vi "AudioTest.Compare Plot to Limit, Get Margin.vi"(8 "error in (no error)":errorcluster, 10 "Plot Limit":T1, 11 "Plot Data":T1) -> (0 "error out":errorcluster, 3 "Margin":dbl)   [LabVIEW 2018]
uses:
  TypeDefs/AudioTest.Result Plot Data.ctl
panel:
  out "Freq":dbl
  out "XY Graph":cluster{"X":dbl[], "Y":dbl[]}[](graph)
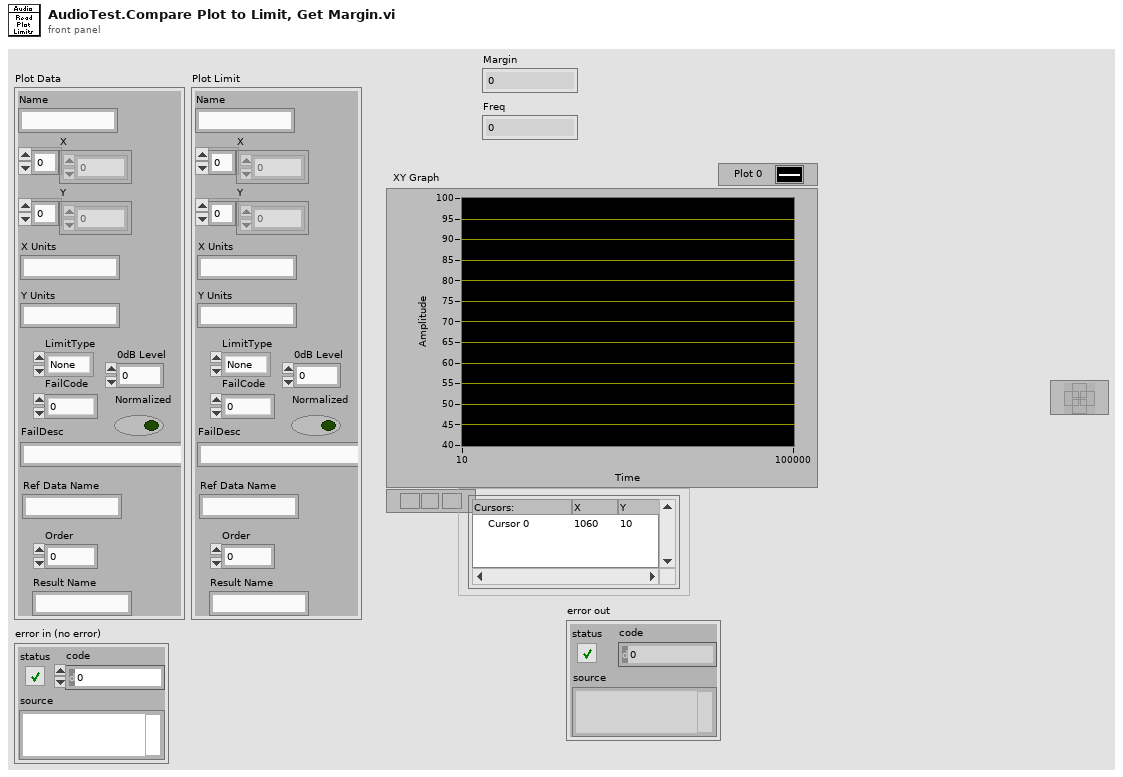
[diagram p1: front panel]
types:
  T1 = typedef "AudioTest.Result Plot Data.ctl" = cluster{"Order":i32, "Name":string, "X":dbl[], "Y":dbl[], "X Units":string, "Y Units":string, "LimitType":enum16{"None", "LL", "UL"}, "FailCode":i32, "FailDesc":string, "Ref Data Name":string, "Result Name":string, "0dB Level":dbl, "Normalized":bool}
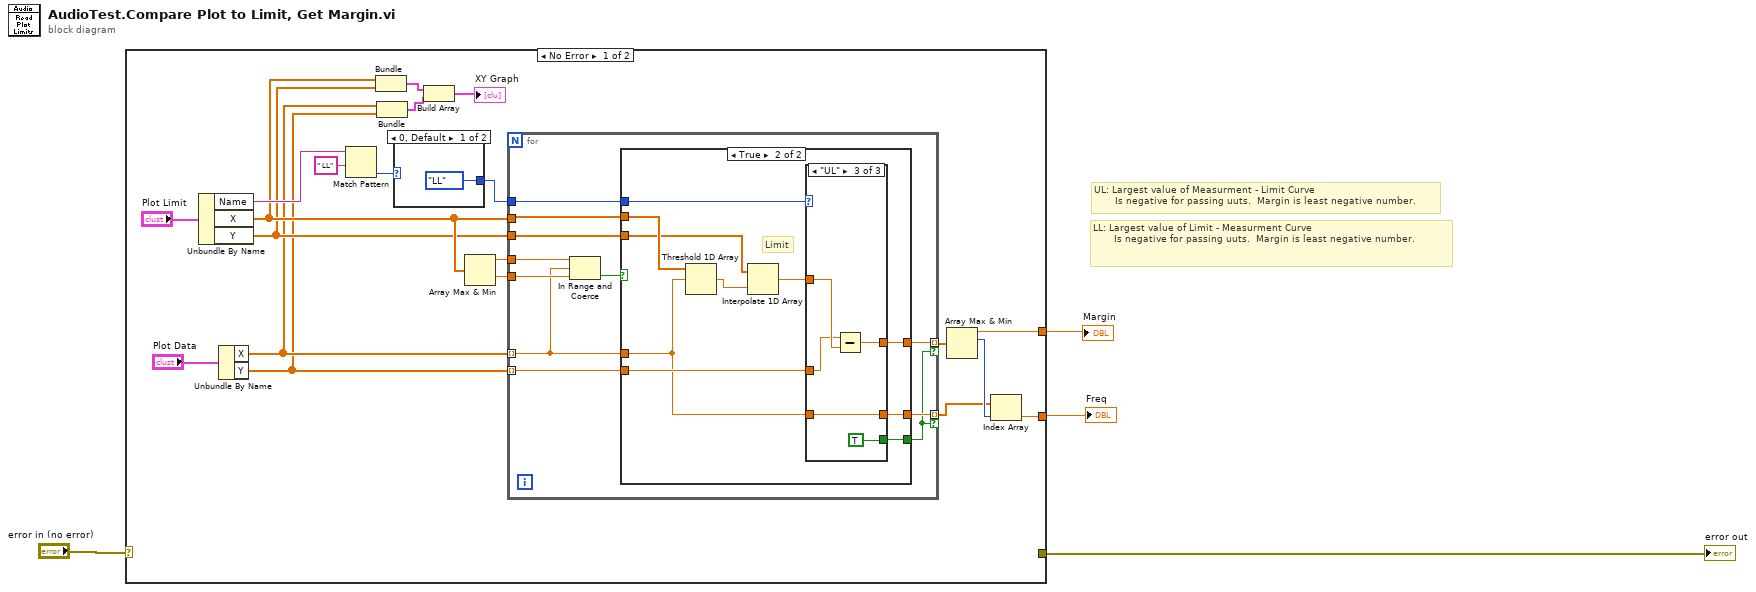
[diagram p0: block diagram]
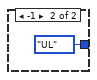
[diagram p2: hidden frame]
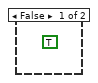
[diagram p3: hidden frame]
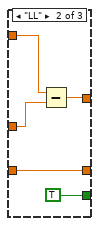
[diagram p5: hidden frame]
diagram:
  # "LL: Largest value of Limit - Measurment Curve\n       Is negative for passing uuts.  Margin is least negative number."
  # "UL: Largest value of Measurment - Limit Curve\n       Is negative for passing uuts.  Margin is least negative number."
  n1 = case shown="No Error" "error in (no error)" {
    selector: "error in (no error)" -> [_ w58]
    tunnel: [_ w58] -> w3
    tunnel: [w19 _] -> w2
    tunnel: [w5 _] -> w1
    frame No Error {
      n2 = Unbundle By Name("Plot Limit") -> ("Name"=w18:string, "X"=w14:dbl[], "Y"=w13:dbl[])
      n3 = Unbundle By Name("Plot Data") -> ("X"=w12:dbl[], "Y"=w11:dbl[])
      n4 = Match Pattern(string=w18, regular expression=" LL") -> (offset past match=w16:i32)  [unwired: 1 in, 3 out]
      n5 = Bundle("X"=w14, "Y"=w13) -> (w10:cluster{"X":dbl[], "Y":dbl[]})  [unwired: 1 in]
      n6 = Bundle("X"=w12, "Y"=w11) -> (w9:cluster{"X":dbl[], "Y":dbl[]})  [unwired: 1 in]
      n7 = case shown="0, Default" w16 {
        tunnel: [enum16{"None", "LL", "UL"}."LL" ("LimitType") enum16{"None", "LL", "UL"}."UL" ("LimitType")] -> w15
        frame 0, Default {
        }
        frame -1 {
        }
      }
      n8 = Build Array(w10, w9) -> (→"XY Graph":cluster{"X":dbl[], "Y":dbl[]}[])
      n9 = Array Max & Min(array=w14) -> (max value=w22:dbl, min value=w21:dbl)  [unwired: 2 out]
      n10 = for {
        tunnel: w14 -> [w32]
        tunnel: w13 -> [w31]
        tunnel: w12 -> [w33] mode=indexing
        tunnel: w11 -> [w35] mode=indexing
        tunnel: w22 -> [w37]
        tunnel: w21 -> [w36]
        tunnel: w15 -> [w30]
        tunnel: [w29] -> w6 mode=indexing if=w27
        tunnel: [w28] -> w20 mode=indexing if=w27
        n11 = In Range and Coerce(upper limit=w37, x=w33, lower limit=w36) -> (In Range?=w34:bool)  [unwired: 1 out]
        n12 = case shown="True" w34 {
          tunnel: w35 -> [_ w43]
          tunnel: w33 -> [_ w41]
          tunnel: w32 -> [_ w47]
          tunnel: w31 -> [_ w45]
          tunnel: w30 -> [_ w44]
          tunnel: [_ w40] -> w29
          tunnel: [_ w39] -> w28
          tunnel: [_ w38] -> w27
          frame False {
            (unwired) TRUE
          }
          frame True {
            # "Limit"
            n13 = Threshold 1D Array(2:w41, 3:w47) -> (0:w46:dbl)  [unwired: 1 in]
            n14 = Interpolate 1D Array(1:w46, 2:w45) -> (0:w42:dbl)
            n15 = case shown="\"UL\"" w44 {
              tunnel: w42 -> [_ w51 w55]
              tunnel: w43 -> [_ w50 w54]
              tunnel: w41 -> [_ w52 w57]
              tunnel: [_ w52 w57] -> w40
              tunnel: [_ w48 w56] -> w39
              tunnel: [_ TRUE TRUE] -> w38
              frame "None", Default {
              }
              frame "LL" {
                n16 = Subtract(x=w51, y=w50) -> (x-y=w48:dbl)
              }
              frame "UL" {
                n17 = Subtract(x=w54, y=w55) -> (x-y=w56:dbl)
              }
            }
          }
        }
      }
      n18 = Array Max & Min(array=w20) -> (max value=w19:dbl, max index (indices)=w7:i32)  [unwired: 2 out]
      n19 = Index Array(array=w6, index=w7) -> (element=w5:dbl)
    }
    frame Error {
      (unwired) u32 16777216
    }
  }
  "error out" <- w3
  "Margin" <- w2
  "Freq" <- w1
